vi "Chirp_DC_WaitStable.vi"(8 "error in (no error)":errorcluster, 11 "ChirpEIS in":refnum<class "ChirpEIS.lvclass">) -> (0 "error out":errorcluster, 1 "data":dynamicdata(graph), 2 "logical AND":bool, 3 "ChirpEIS out":refnum<class "ChirpEIS.lvclass">)   [LabVIEW 2014, in "ChirpEIS.lvclass"]
uses:
  ChirpEIS.lvclass
  ChirpEIS.lvclass/ChirpEIS.ctl
  <vilib>/Analysis/baseanly.llb/Mean (DBL).vi
  <vilib>/Analysis/NI_AALBase.lvlib
  <vilib>/measure/NI_MABase.lvlib
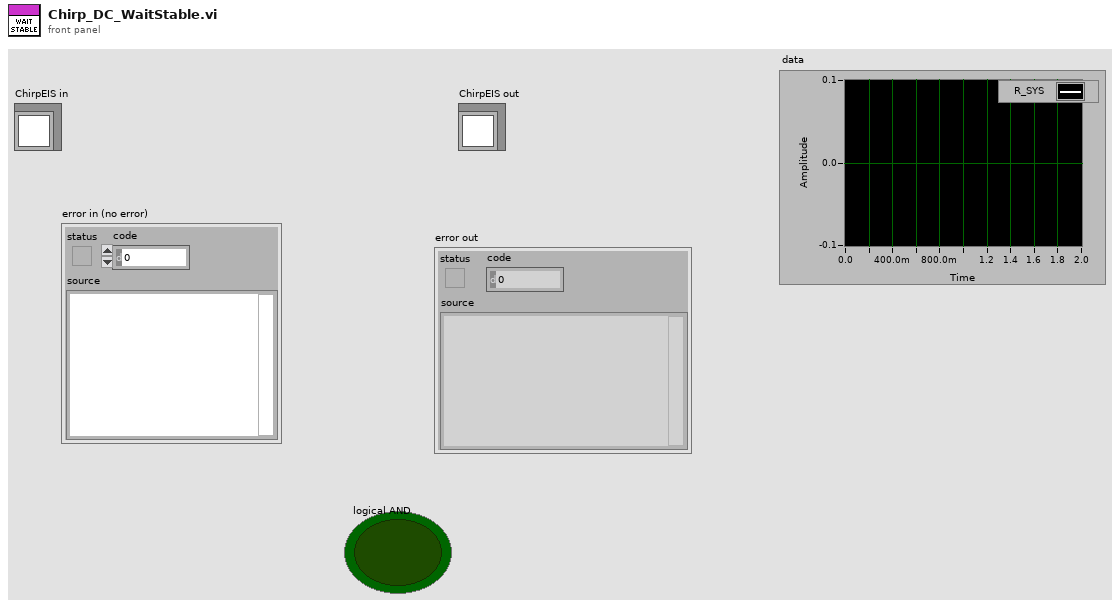
[diagram p1: front panel]
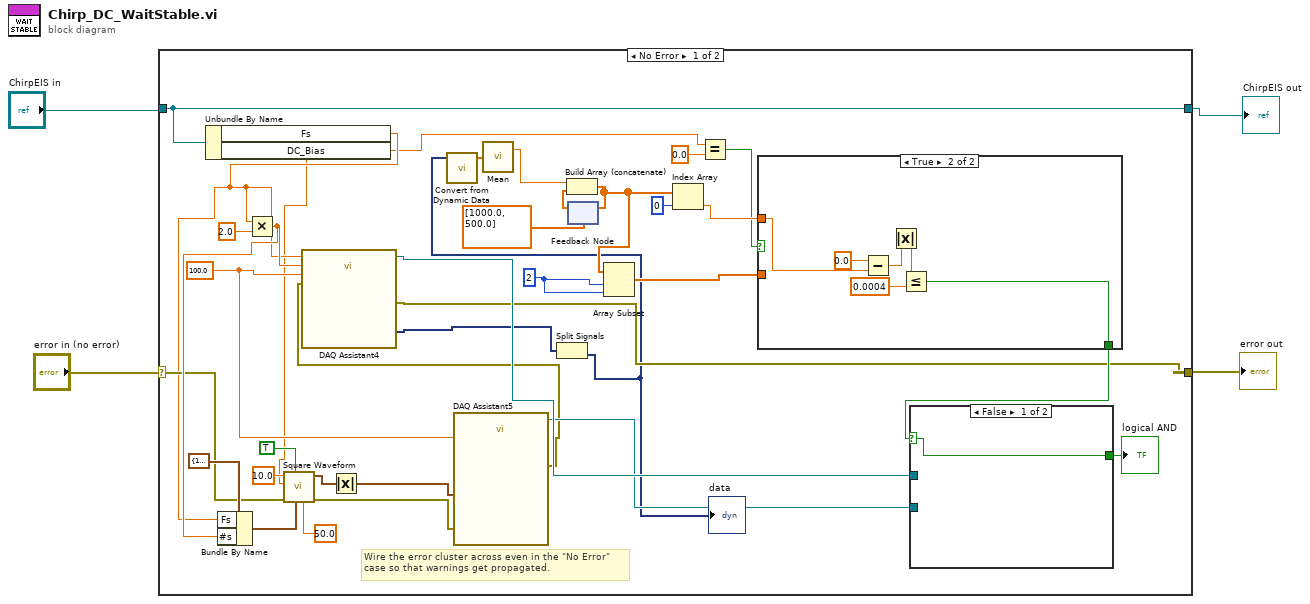
[diagram p0: block diagram]
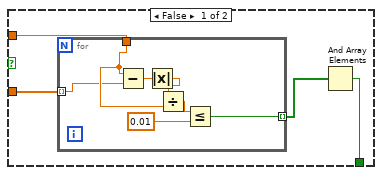
[diagram p2: hidden frame]
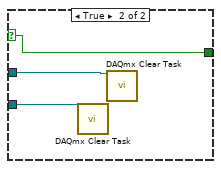
[diagram p3: hidden frame]
diagram:
  n1 = case shown="No Error" "error in (no error)" {
    selector: "error in (no error)" -> [w14 w61]
    tunnel: [w15 w61] -> w1
    tunnel: [w30 w60] -> w3
    tunnel: "ChirpEIS in" -> [w30 w60]
    frame No Error {
      w24 = 100.0 ("timeout (s)")
      w37 = 2 ("y")
      # "Wire the error cluster across even in the \"No Error\"\ncase so that warnings get propagated."
      n2 = Unbundle By Name(w30) -> ("Fs"=w8:dbl, "DC_Bias"=w7:dbl)
      n3 = Multiply(x=w8, y=2.0) -> (x*y=w20:dbl)
      n4 = Bundle By Name(cluster=cluster{"Fs":dbl, "#s":dbl} {"Fs"=1000.0, "#s"=1000.0} ("sampling info"), "Fs"=w8, "#s"=w20) -> (w19:cluster{"Fs":dbl, "#s":dbl})
      n5 = call <vilib>:"Square Waveform.vi"("duty cycle (%)"=50.0, "sampling info"=w19, "reset signal"=TRUE, "error in (no error)"=w14, "amplitude"=w7, "frequency"=10.0) -> ("error out"=w13:errorcluster, "signal out"=w18:waveform(dbl))  [unwired: 4 in]
      n6 = Absolute Value(x=w18) -> (abs(x)=w11:waveform(dbl))
      n7 = call "DAQ Assistant5"("data"=w11, "timeout (s)"=w24, "error in"=w13) -> ("task out"=w16:refnum<k21>, "error out"=w12:errorcluster)  [unwired: 14 in, 1 out]
      n8 = call "DAQ Assistant4"("rate"=w8, "number of samples"=w20, "timeout (s)"=w24, "error in"=w12) -> ("task out"=w27:refnum<k21>, "data"=w17:dynamicdata, "error out"=w15:errorcluster)  [unwired: 13 in]
      n9 = Split Signals(w17) -> (w9:dynamicdata)  [unwired: 2 in, 1 out]
      "data" <- w9
      n10 = call "Convert from Dynamic Data"("Dynamic Data Type"=w9) -> ("Array"=w26:dbl[])  [unwired: 3 in]
      n11 = call-poly <vilib>:"Mean.vi"("X"=w26) -> ("mean"=w31:dbl)  [unwired: 1 out]
      n12 = feedback #1(dbl[] [1000.0, 500.0]) -> (w32:dbl[])
      n13 = Build Array (concatenate)(w31, w32) -> (w35:dbl[])
      n14 = feedback-in #1(w35) -> ()
      n15 = Array Subset(array=w35, index=w37, length=w37) -> (w36:dbl[])
      n16 = Index Array(array=w35, index=0) -> (element=w34:dbl)
      n17 = Equal?(x=w7, y=0.0) -> (x = y?=w5:bool)
      n18 = case shown="True" w5 {
        tunnel: w36 -> [w42 _]
        tunnel: w34 -> [w41 w51]
        tunnel: [w40 w50] -> w29
        frame False {
          n19 = for {
            tunnel: w41 -> [w47]
            tunnel: w42 -> [w44] mode=indexing
            tunnel: [w43] -> w39 mode=indexing
            n20 = Subtract(x=w47, y=w44) -> (x-y=w49:dbl)
            n21 = Absolute Value(x=w49) -> (abs(x)=w48:dbl)
            n22 = Divide(x=w48, y=w47) -> (x/y=w46:dbl)
            n23 = Less Or Equal?(x=w46, y=0.01) -> (x <= y?=w43:bool)
          }
          n24 = And Array Elements(Boolean array=w39) -> (logical AND=w40:bool)
        }
        frame True {
          n25 = Subtract(x=0.0, y=w51) -> (x-y=w54:dbl)
          n26 = Absolute Value(x=w54) -> (abs(x)=w55:dbl)
          n27 = Less Or Equal?(x=w55, y=0.0004) -> (x <= y?=w50:bool)
        }
      }
      n28 = case shown="False" w29 {
        selector: w29 -> [w56 w58]
        tunnel: w27 -> [_ w59]
        tunnel: [w56 w58] -> w25
        tunnel: w16 -> [_ w57]
        frame False {
        }
        frame True {
          n29 = call <vilib>:"DAQmx Clear Task.vi"("task in"=w57) -> ()  [unwired: 14 in, 1 out]
          n30 = call <vilib>:"DAQmx Clear Task.vi"("task in"=w59) -> ()  [unwired: 14 in, 1 out]
        }
      }
      "logical AND" <- w25
    }
    frame Error {
    }
  }
  "ChirpEIS out" <- w3
  "error out" <- w1
